vi "dodaj przebieg kursor.vi"(4 "Plot.Y Scale Index":u32, 6 "WaveformGraph in":refnum<vi>, 8 "error in (no error)":errorcluster, 9 "Data":T1, 10 "Pomiarowe OK?":bool, 11 "Przebiegi in":waveform(dbl)[](array[waveform])) -> (0 "error out":errorcluster, 3 "przebiegi out":waveform(dbl)[](array[waveform]))   [LabVIEW 2014]
doc: "Dodaje wykres kursor\njeżeli istnieją dwa kursoty pomiarowe"
uses:
  Kontrolki/GUI/Wysw_kursorow_silver.ctl
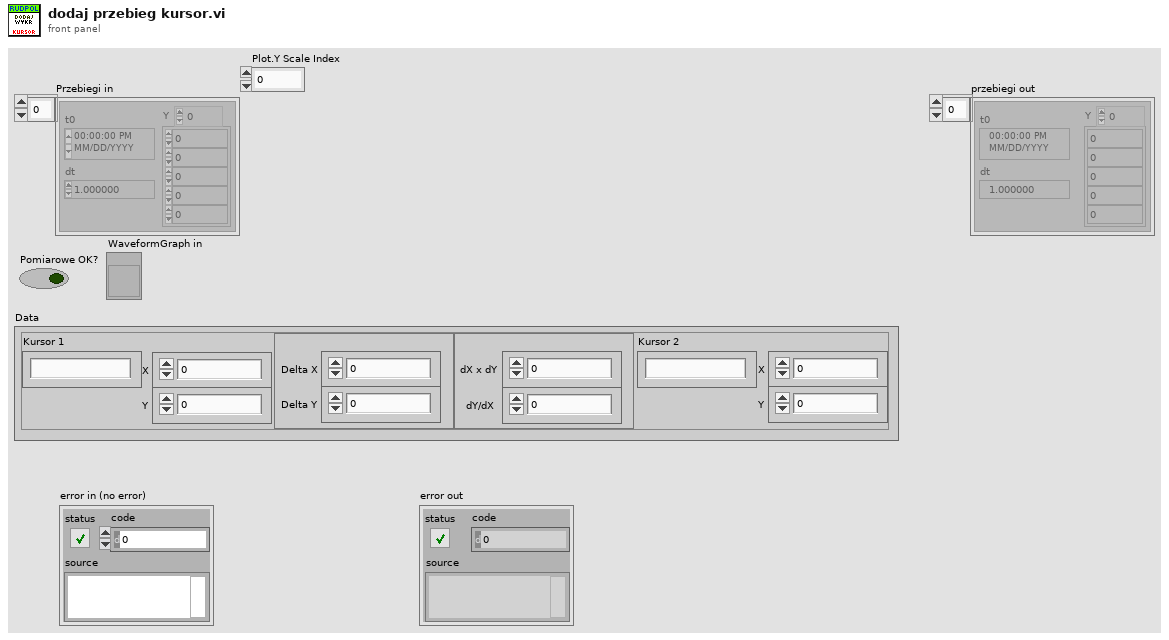
[diagram p1: front panel]
types:
  T1 = typedef "Wysw_kursorow_silver.ctl" = cluster{"Nazwa.1":string, "Nazwa.2":string, "Pos.X1":dbl, "Pos.Y1":dbl, "Delta.X":dbl, "Delta.Y":dbl, "Pos.X2":dbl, "Pos.Y2":dbl, "iloczyn dXY":dbl, "IlorazdYX":dbl}
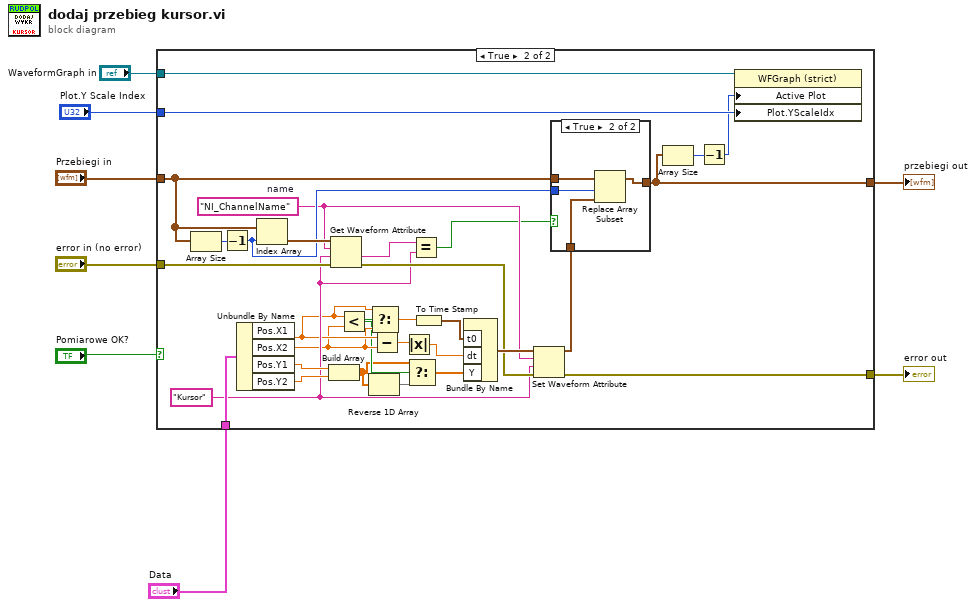
[diagram p0: block diagram]
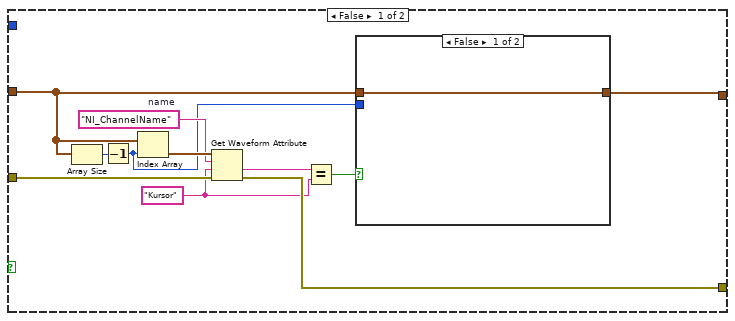
[diagram p2: hidden frame]
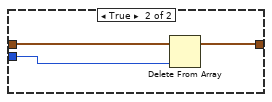
[diagram p3: hidden frame]
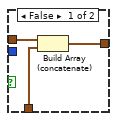
[diagram p4: hidden frame]
diagram:
  n1 = case shown="True" "Pomiarowe OK?" {
    tunnel: "Data" -> [_ w54]
    tunnel: "Przebiegi in" -> [w14 w46]
    tunnel: [w12 w26] -> w8
    tunnel: "error in (no error)" -> [w16 w45]
    tunnel: [w15 w43] -> w3
    tunnel: "WaveformGraph in" -> [_ w28]
    tunnel: "Plot.Y Scale Index" -> [_ w27]
    frame False {
      w10 = "Kursor" ("name")
      w17 = "NI_ChannelName"  # name
      n2 = Array Size(array=w14) -> (size(s)=w19:i32)
      n3 = Decrement(x=w19) -> (x-1=w13:i32)
      n4 = Index Array(array=w14, index=w13) -> (element=w18:waveform(dbl))
      n5 = Get Waveform Attribute(4:w16, 5:w10, 6:w17, 7:w18) -> (0:w15:errorcluster, 1:w11:string)  [unwired: 2 out]
      n6 = Equal?(x=w11, y=w10) -> (x = y?=w9:bool)
      n7 = case shown="False" w9 {
        tunnel: w14 -> [w20 w23]
        tunnel: w13 -> [_ w21]
        tunnel: [w20 w22] -> w12
        frame False {
        }
        frame True {
          n8 = Delete From Array(array=w23, index=w21) -> (array with subset deleted=w22:waveform(dbl)[])  [unwired: 1 in, 1 out]
        }
      }
    }
    frame True {
      w39 = "Kursor" ("name")
      w41 = "NI_ChannelName"  # name
      n9 = Array Size(array=w46) -> (size(s)=w48:i32)
      n10 = Decrement(x=w48) -> (x-1=w42:i32)
      n11 = Unbundle By Name(w54) -> ("Pos.X1"=w36:dbl, "Pos.X2"=w35:dbl, "Pos.Y1"=w53:dbl, "Pos.Y2"=w52:dbl)
      n12 = Index Array(array=w46, index=w42) -> (element=w47:waveform(dbl))
      n13 = Build Array(w53, w52) -> (w30:dbl[])
      n14 = Get Waveform Attribute(4:w45, 5:w39, 6:w41, 7:w47) -> (0:w44:errorcluster, 1:w40:string)  [unwired: 2 out]
      n15 = Less?(x=w36, y=w35) -> (x < y?=w32:bool)
      n16 = Reverse 1D Array(array=w30) -> (reversed array=w29:dbl[])
      n17 = Select(t=w36, s=w32, f=w35) -> (s? t:f=w34:dbl)
      n18 = Subtract(x=w36, y=w35) -> (x-y=w33:dbl)
      n19 = Absolute Value(x=w33) -> (abs(x)=w37:dbl)
      n20 = Select(t=w30, s=w32, f=w29) -> (s? t:f=w31:dbl[])
      n21 = Equal?(x=w40, y=w39) -> (x = y?=w38:bool)
      n22 = To Time Stamp(1:w34) -> (0:w51:timestamp)
      n23 = Bundle By Name("t0"=w51, "dt"=w37, "Y"=w31) -> (w50:waveform(dbl))  [unwired: 1 in]
      n24 = Set Waveform Attribute(4:w44, 5:w39, 6:w41, 7:w50) -> (0:w43:errorcluster, 3:w49:waveform(dbl))  [unwired: 1 out]
      n25 = case shown="True" w38 {
        tunnel: [w57 w61] -> w26
        tunnel: w49 -> [w56 w59]
        tunnel: w46 -> [w55 w58]
        tunnel: w42 -> [_ w60]
        frame False {
          n26 = Build Array (concatenate)(w55, w56) -> (w57:waveform(dbl)[])
        }
        frame True {
          n27 = Replace Array Subset(array=w58, new element=w59, index=w60) -> (w61:waveform(dbl)[])
        }
      }
      n28 = Array Size(array=w26) -> (size(s)=w25:i32)
      n29 = Decrement(x=w25) -> (x-1=w24:i32)
      n30 = property class="WFGraph (strict)"(reference=w28, "Active Plot"=w24, "Plot.YScaleIdx"=w27) -> ()  [unwired: 1 in, 2 out]
    }
  }
  "przebiegi out" <- w8
  "error out" <- w3
